vi "Configure Measurement.vi"(6 "Manual Range (1)":dbl=1.0, 7 "Auto Range (T: Enable)":bool=TRUE, 8 "error in (no error)":errorcluster, 9 "Channel List(\"\")":string, 10 "Function (0: Voltage DC)":i32(ring) items=["Voltage DC", "Voltage AC", "Current DC", "Current AC", "Resistance", "4-wire Resistance", "Diode", "Capacitance", "Temperature", "Continuity", "Frequency", "Period", "Voltage Ratio", "Digitize Voltage", "Digitize Current"], 11 "VISA resource name":refnum<visa-resource-name>) -> (0 "error out":errorcluster, 3 "VISA resource name out":refnum<visa-resource-name>)   [LabVIEW 2024, in "Keithley DMM6500 DAQ6500 Series.lvlib"]
doc: "Configures the measurement. Function, auto range, channel list and measure range."
uses:
  Keithley DMM6500 DAQ6500 Series.lvlib
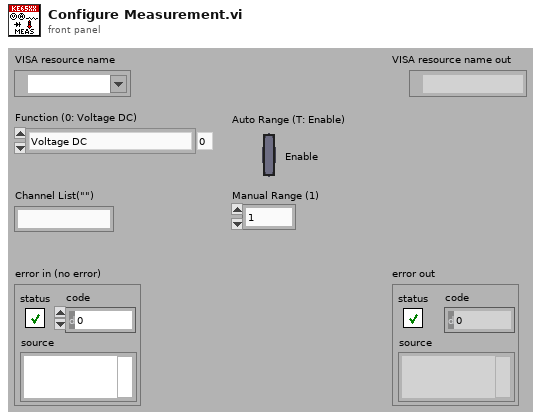
[diagram p1: front panel]
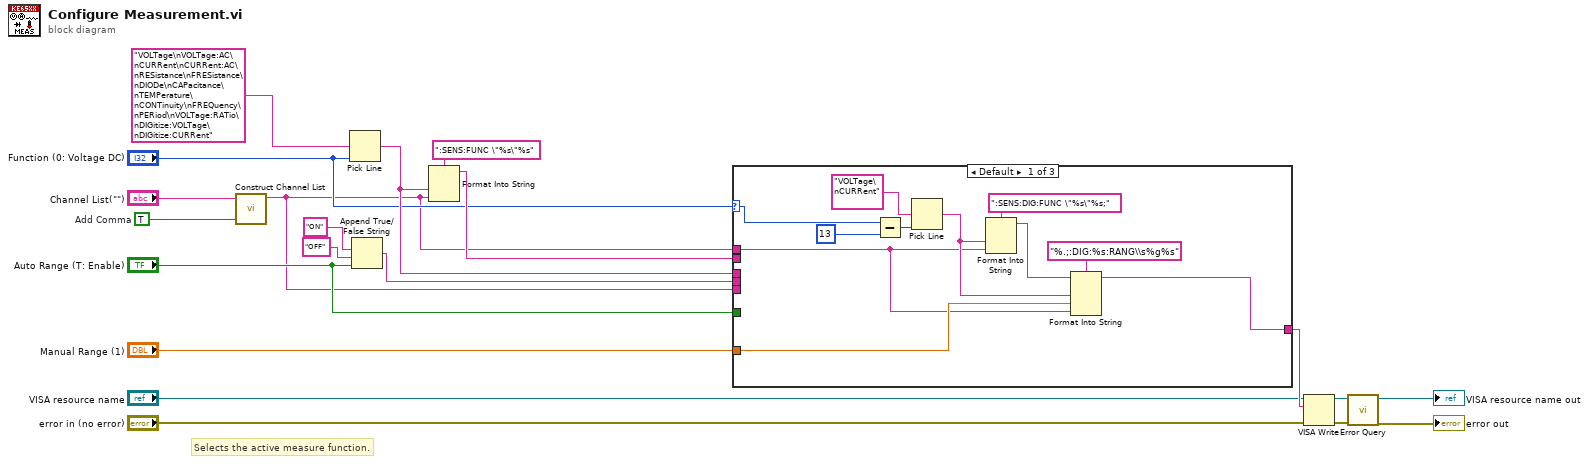
[diagram p0: block diagram]
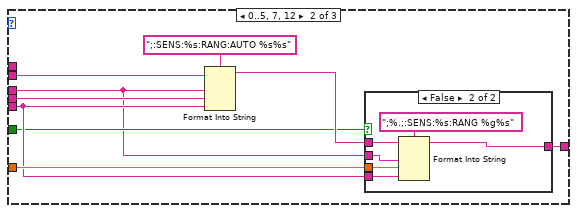
[diagram p2: hidden frame]
diagram:
  w2 = TRUE  # Add Comma
  # "Selects the active measure function."
  n1 = call "Construct Channel List.vi"("Add Comma (True)"=w2, "Channel List"="Channel List(\"\")") -> ("Channel List String"=w1:string)  [unwired: 1 in]
  n2 = Pick Line(multi-line string="VOLTage\nVOLTage:AC\nCURRent\nCURRent:AC\nRESistance\nFRESistance\nDIODe\nCAPacitance\nTEMPerature\nCONTinuity\nFREQuency\nPERiod\nVOLTage:RATio\nDIGitize:VOLTage\nDIGitize:CURRent", line index="Function (0: Voltage DC)") -> (output string=w4:string)  [unwired: 1 in]
  n3 = Append True/False String(1:"Auto Range (T: Enable)", 2:"OFF", 3:"ON") -> (0:w16:string)  [unwired: 1 in]
  n4 = Format Into String(format string=":SENS:FUNC \"%s\"%s", w4, w1) -> (resulting string=w17:string)  [unwired: 2 in, 1 out]
  n5 = case shown="Default" "Function (0: Voltage DC)" {
    selector: "Function (0: Voltage DC)" -> [w28 _ _]
    tunnel: w17 -> [_ w40 w48]
    tunnel: w16 -> [_ w39 _]
    tunnel: "Manual Range (1)" -> [w24 w37 _]
    tunnel: [w21 w36 w48] -> w14
    tunnel: w1 -> [_ w35 _]
    tunnel: "Auto Range (T: Enable)" -> [_ w34 _]
    tunnel: w4 -> [_ w33 _]
    tunnel: w1 -> [w22 _ _]
    frame Default {
      n6 = Subtract(x=w28, y=13) -> (x-y=w29:i32)
      n7 = Pick Line(multi-line string="VOLTage\nCURRent", line index=w29) -> (output string=w23:string)  [unwired: 1 in]
      n8 = Format Into String(format string=":SENS:DIG:FUNC \"%s\"%s;", w23, w22) -> (resulting string=w25:string)  [unwired: 2 in, 1 out]
      n9 = Format Into String(format string="%.;:DIG:%s:RANG\\s%g%s", initial string=w25, w23, w24, w22) -> (resulting string=w21:string)  [unwired: 1 in, 1 out]
    }
    frame 0..5, 7, 12 {
      n10 = Format Into String(format string=";:SENS:%s:RANG:AUTO %s%s", initial string=w40, w33, w39, w35) -> (resulting string=w38:string)  [unwired: 1 in, 1 out]
      n11 = case shown="False" w34 {
        tunnel: w38 -> [w41 w47]
        tunnel: w37 -> [_ w45]
        tunnel: [w41 w44] -> w36
        tunnel: w35 -> [_ w43]
        tunnel: w33 -> [_ w42]
        frame True {
        }
        frame False {
          n12 = Format Into String(format string=";%.;:SENS:%s:RANG %g%s", initial string=w47, w42, w45, w43) -> (resulting string=w44:string)  [unwired: 1 in, 1 out]
        }
      }
    }
    frame 6, 8..11 {
    }
  }
  n13 = VISA Write(VISA resource name="VISA resource name", write buffer=w14, error in (no error)="error in (no error)") -> (VISA resource name out=w11:refnum<visa-resource-name>, error out=w10:errorcluster)  [unwired: 1 out]
  n14 = call "Error Query.vi"("error in (no error)"=w10, "VISA resource name"=w11) -> ("error out"=→"error out":errorcluster, "VISA resource name out"=→"VISA resource name out":refnum<visa-resource-name>)  [unwired: 6 in, 2 out]
